vi "Round to Zero.vi"(1 "complex":cdb[](array[numeric]) format="%0.2f") -> (0 "result":cdb[](array[numeric]) format="%0.2f")   [LabVIEW 2017, in "NI_PtbyPt.lvlib"]
doc: "Truncates the extremely small complex value to zero."
uses:
  <vilib>/ptbypt/NI_PtbyPt.lvlib
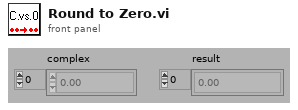
[diagram p1: front panel]
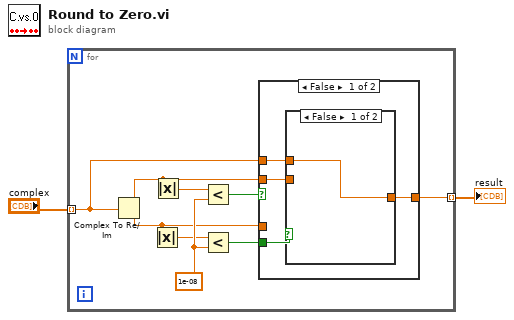
[diagram p0: block diagram]
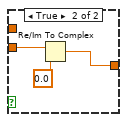
[diagram p2: hidden frame]
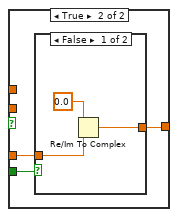
[diagram p3: hidden frame]
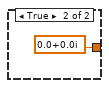
[diagram p4: hidden frame]
diagram:
  n1 = for {
    tunnel: "complex" -> [w8] mode=indexing
    tunnel: [w7] -> w1 mode=indexing
    w11 = 1e-08
    n2 = Complex To Re/Im(x + iy=w8) -> (x=w6:dbl, y=w3:dbl)
    n3 = Absolute Value(x=w3) -> (abs(x)=w4:dbl)
    n4 = Absolute Value(x=w6) -> (abs(x)=w5:dbl)
    n5 = Less?(x=w5, y=w11) -> (x < y?=w10:bool)
    n6 = Less?(x=w4, y=w11) -> (x < y?=w9:bool)
    n7 = case shown="False" w10 {
      tunnel: w9 -> [w15 w22]
      tunnel: w8 -> [w14 _]
      tunnel: [w13 w21] -> w7
      tunnel: w3 -> [_ w20]
      tunnel: w6 -> [w12 _]
      frame False {
        n8 = case shown="False" w15 {
          tunnel: w14 -> [w16 _]
          tunnel: [w16 w17] -> w13
          tunnel: w12 -> [_ w18]
          frame False {
          }
          frame True {
            n9 = Re/Im To Complex(1:0.0, 2:w18) -> (0:w17:cdb)
          }
        }
      }
      frame True {
        n10 = case shown="False" w22 {
          tunnel: [w23 cdb 0.0+0.0i] -> w21
          tunnel: w20 -> [w24 _]
          frame False {
            n11 = Re/Im To Complex(1:w24, 2:0.0) -> (0:w23:cdb)
          }
          frame True {
          }
        }
      }
    }
  }
  "result" <- w1
